vi "junk.vi"() -> ()   [LabVIEW 2013]
panel:
  out "Tab Control 2":T1(tab)
  in  "Tab Control":T1(tab)
  out "Waveform Graph 2":waveform(dbl)(graph)
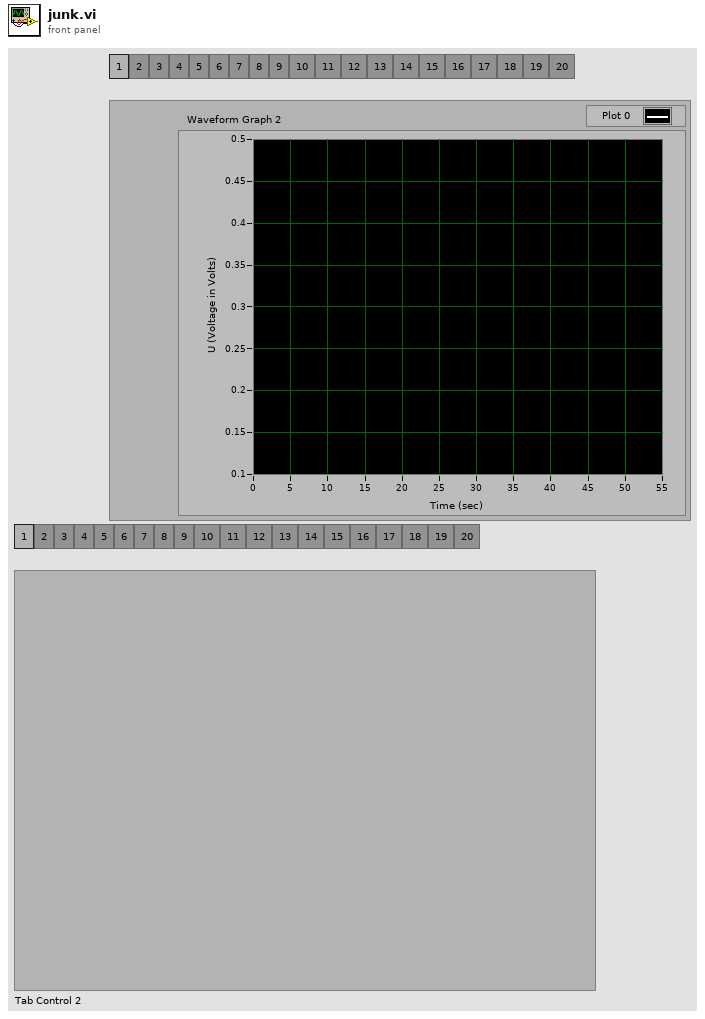
[diagram p1: front panel]
types:
  T1 = enum32{"1", "2", "3", "4", "5", "6", "7", "8", "9", "10", "11", "12", "13", "14", "15", "16", "17", "18", "19", "20"}
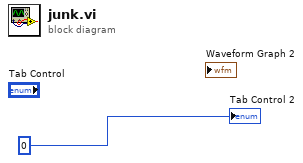
[diagram p0: block diagram]
diagram:
  "Tab Control 2" <- 0
